vi "Decode Data.vi"(8 "Errors In":T1, 10 "Time Stamp":timestamp, 11 "Data Array":string[](array[string])) -> (0 "Errors Out":T1, 3 "logData Out":T2)   [LabVIEW 2014]
doc: "Decode hex data obtained from inverter boards into decimal measurements. DC bus voltage, current RMS, motor power, temp."
uses:
  TypeDefs/Errors.ctl
panel:
  in  "logData In":T3
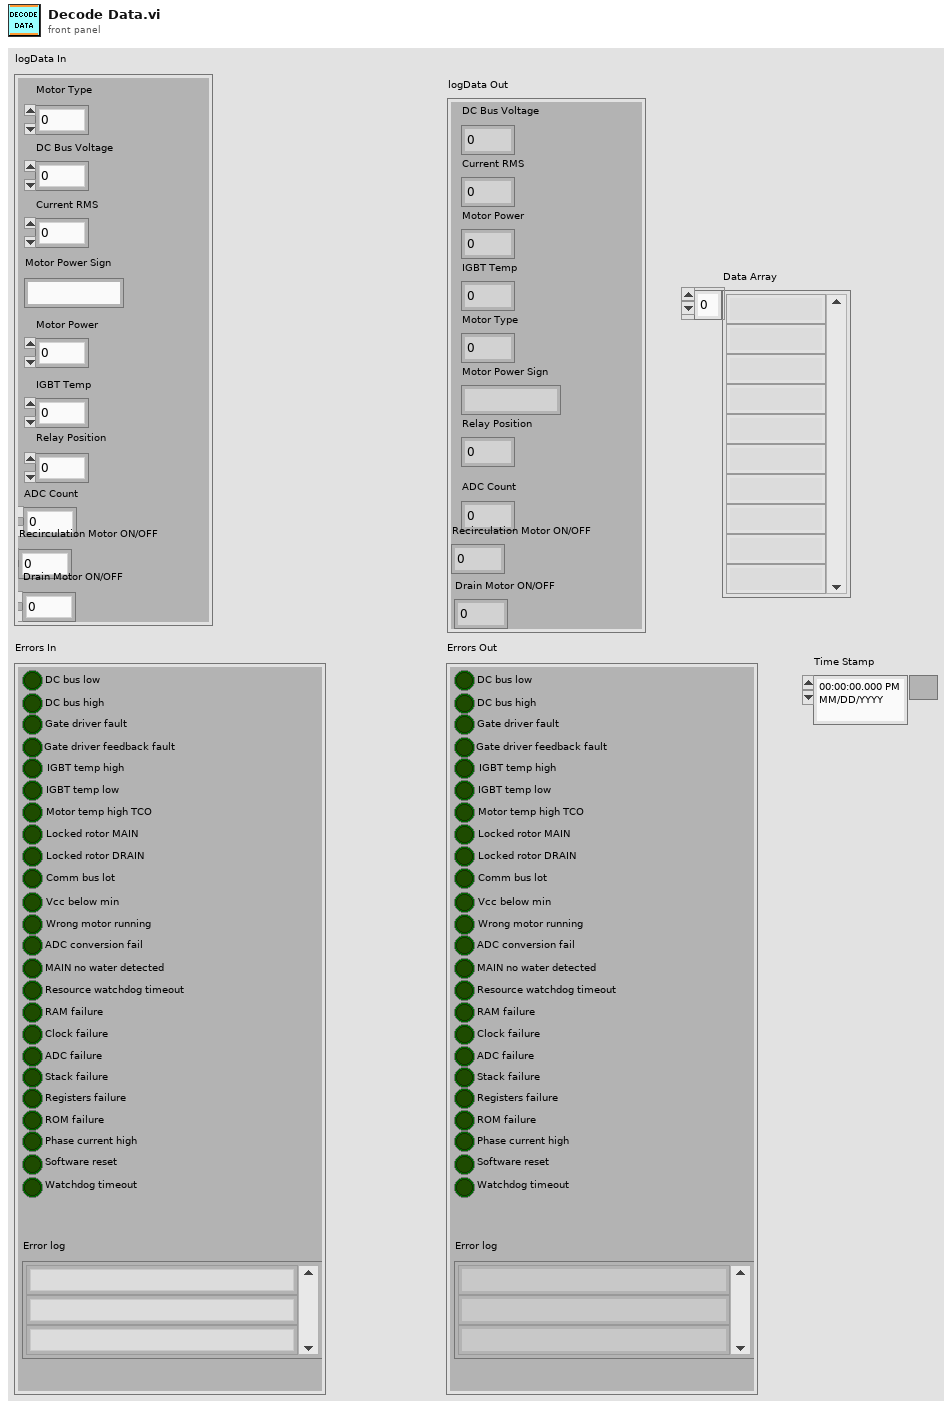
[diagram p1: front panel]
types:
  T1 = typedef "Errors.ctl" = cluster{"DC bus low":bool, "DC bus high":bool, "Gate driver fault":bool, "Gate driver feedback fault":bool, "IGBT temp high":bool, "IGBT temp low":bool, "Motor temp high TCO":bool, "Locked rotor MAIN":bool, "Locked rotor DRAIN":bool, "Comm bus lot":bool, "Vcc below min":bool, "Wrong motor running":bool, "ADC conversion fail":bool, "MAIN no water detected":bool, "Resource watchdog timeout":bool, "RAM failure":bool, "Clock failure":bool, "ADC failure":bool, "Stack failure":bool, "Registers failure":bool, "ROM failure":bool, "Phase current high":bool, "Software reset":bool, "Watchdog timeout":bool, "Error log":string[]}
  T2 = cluster{"DC Bus Voltage":dbl, "Current RMS":dbl, "Motor Power":dbl, "IGBT Temp":u16, "Motor Type":u16, "Motor Power Sign":string, "Relay Position":u16, "ADC Count":dbl, "Recirculation Motor ON/OFF":u16, "Drain Motor ON/OFF":u16}
  T3 = cluster{"DC Bus Voltage":dbl, "Current RMS":dbl, "Motor Power":dbl, "IGBT Temp":u32, "Motor Type":u16, "Motor Power Sign":string, "Relay Position":u16, "ADC Count":dbl, "Recirculation Motor ON/OFF":u32, "Drain Motor ON/OFF":u16}
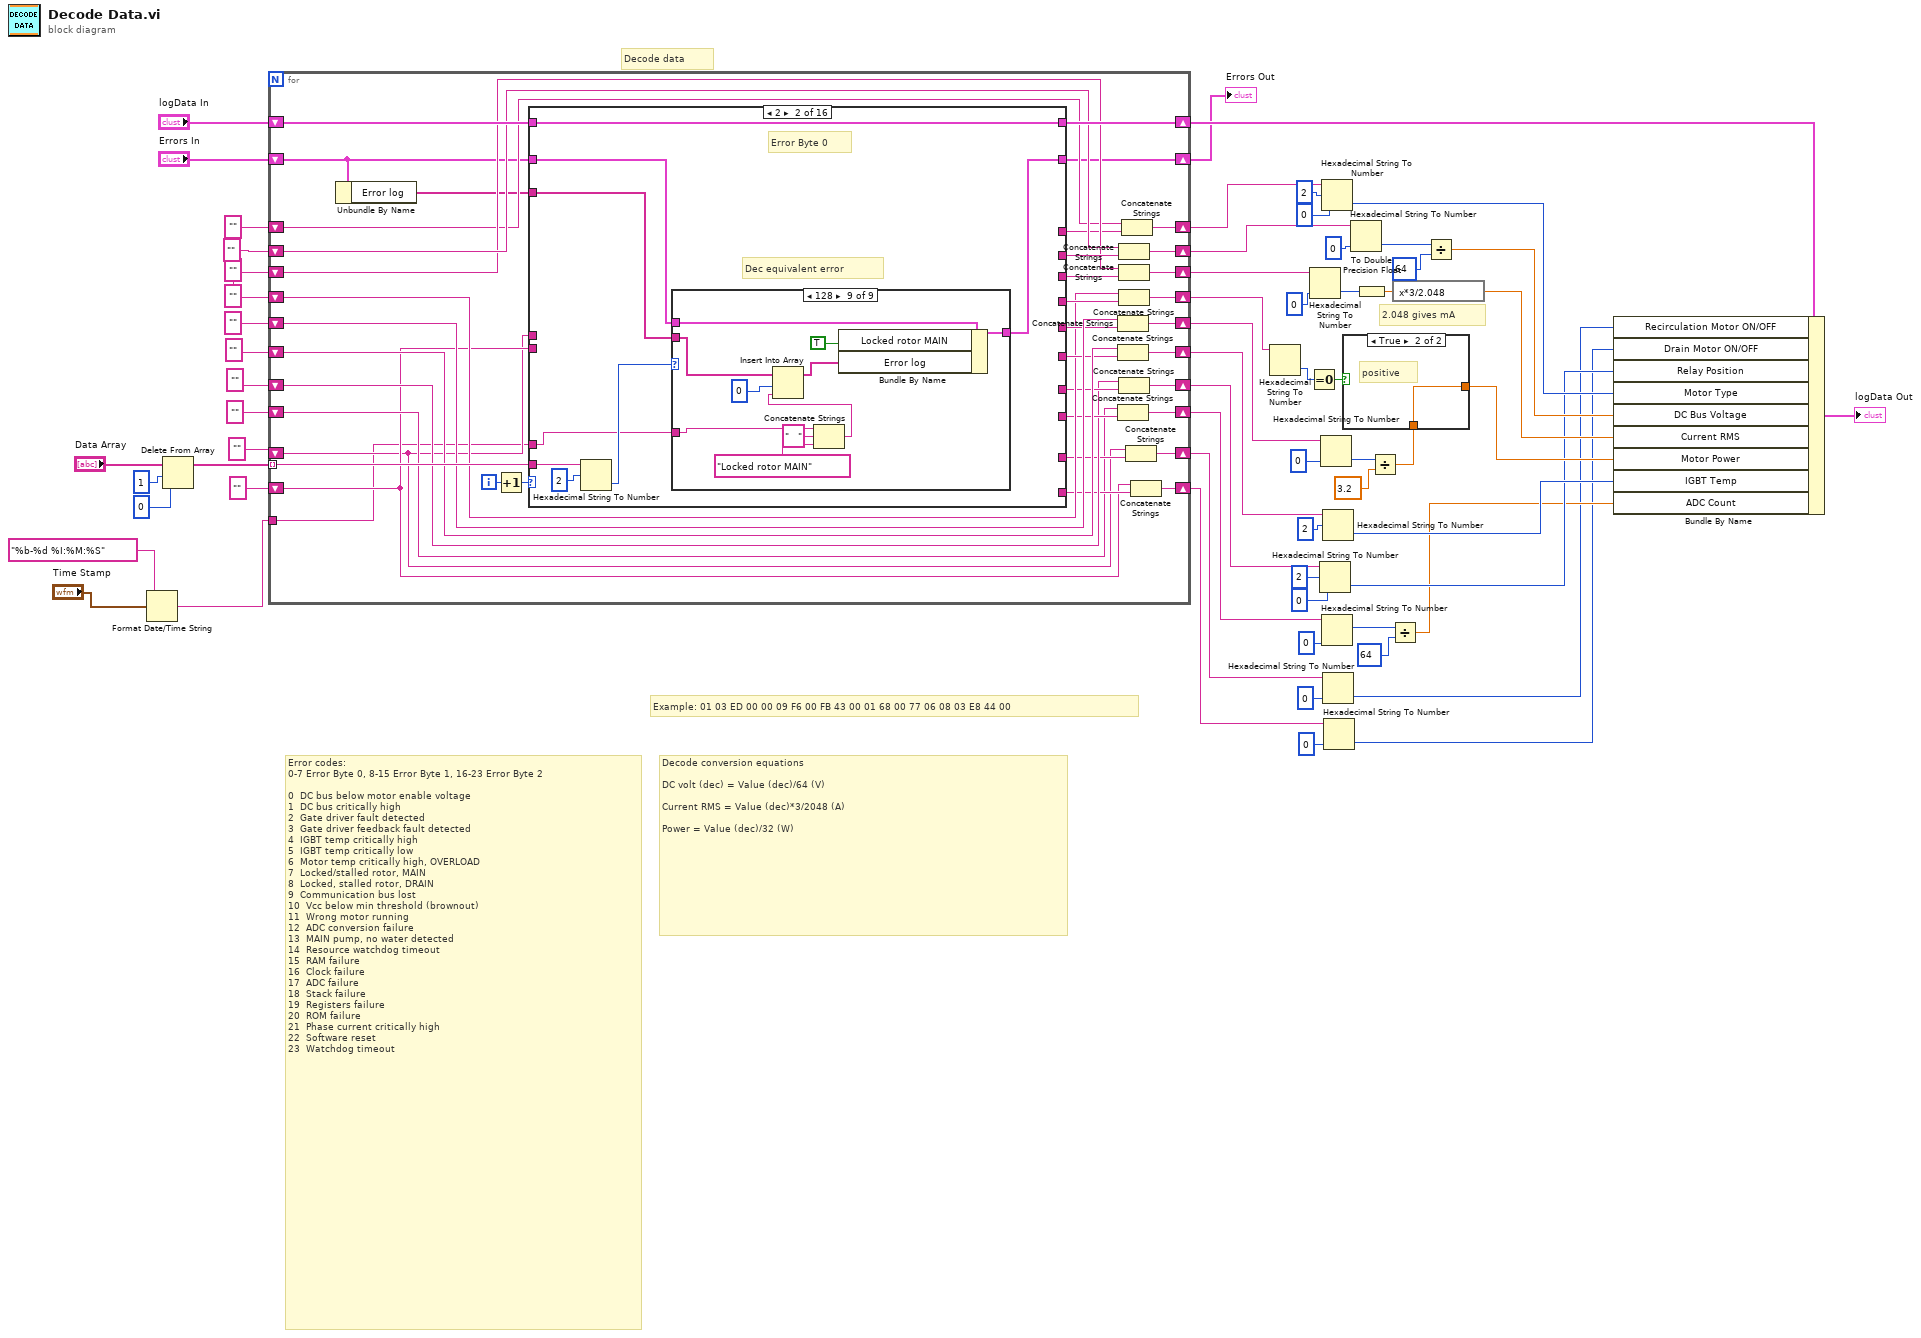
[diagram p0: block diagram]
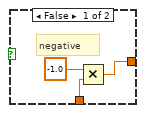
[diagram p2: hidden frame]
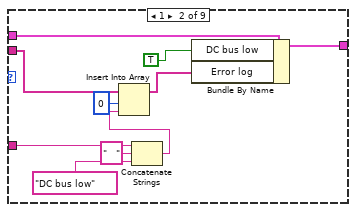
[diagram p5: hidden frame]
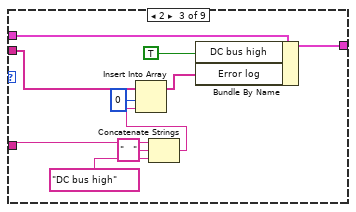
[diagram p6: hidden frame]
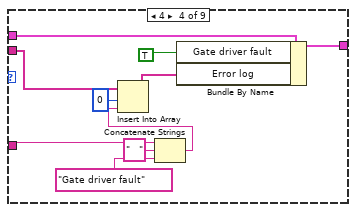
[diagram p7: hidden frame]
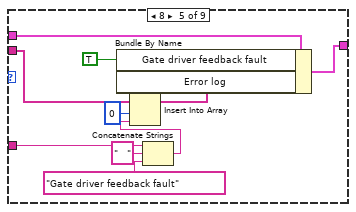
[diagram p8: hidden frame]
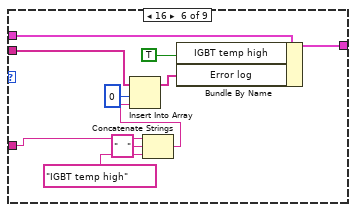
[diagram p9: hidden frame]
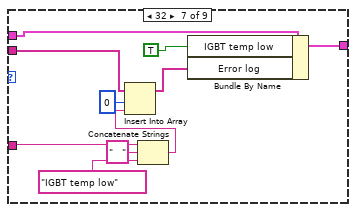
[diagram p10: hidden frame]
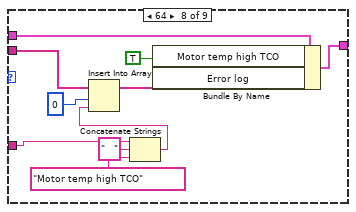
[diagram p11: hidden frame]
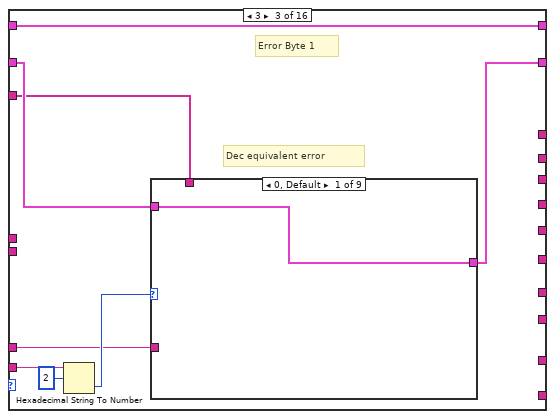
[diagram p12: hidden frame]
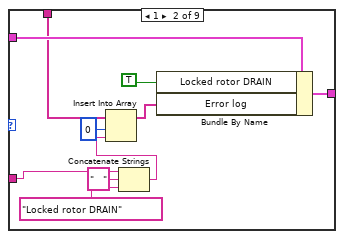
[diagram p13: hidden frame]
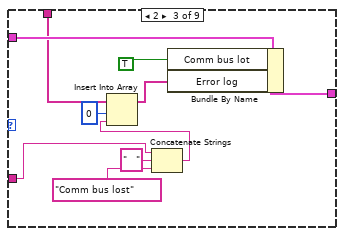
[diagram p14: hidden frame]
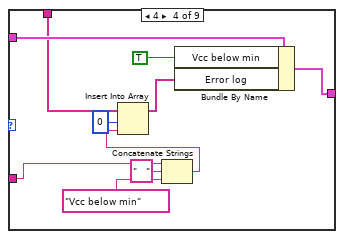
[diagram p15: hidden frame]
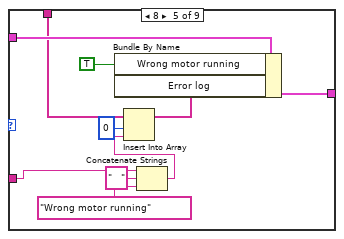
[diagram p16: hidden frame]
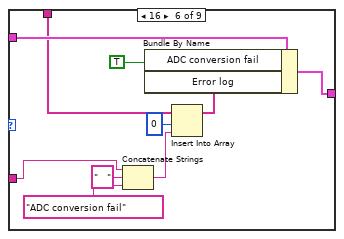
[diagram p17: hidden frame]
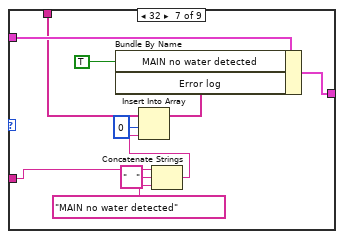
[diagram p18: hidden frame]
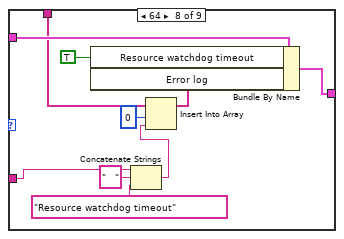
[diagram p19: hidden frame]
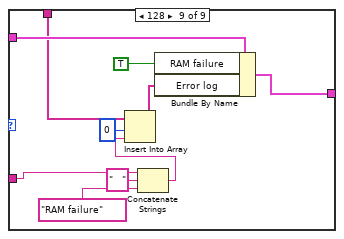
[diagram p20: hidden frame]
diagram:
  # "2.048 gives mA"
  # "Decode conversion equations\n\nDC volt (dec) = Value (dec)/64 (V)\n\nCurrent RMS = Value (dec)*3/2048 (A)\n\nPower = Value (dec)/32 (W)"
  # "Error codes:\n0-7 Error Byte 0, 8-15 Error Byte 1, 16-23 Error Byte 2\n\n0  DC bus below motor enable voltage\n1  DC bus critically high\n2  Gate driver fault detected\n3  Gate driver feedback fault detected\n4  IGBT temp critically high\n5  IGBT temp critically low\n6  Motor temp critically high, OVERLOAD\n7  Locked/stalled rotor, MAIN\n8  Locked, stalled rotor, DRAIN\n9  Communication bus lost\n10  Vcc below min threshold (brownout)\n11  Wrong motor running\n12  ADC conversion failure\n13  MAIN pump, no water detected\n14  Resource watchdog timeout\n15  RAM failure \n16  Clock failure\n17  ADC failure\n18  Stack failure\n19  Registers failure\n20  ROM failure\n21  Phase current critically high\n22  Software reset\n23  Watchdog timeout"
  # "Example: 01 03 ED 00 00 09 F6 00 FB 43 00 01 68 00 77 06 08 03 E8 44 00"
  # "Decode data"
  n1 = Format Date/Time String(time format string (%c)="%b-%d %I:%M:%S", seconds (now)="Time Stamp") -> (date/time string=w1:string)  [unwired: 1 in]
  n2 = Delete From Array(array="Data Array", length=1, index=0) -> (array with subset deleted=w4:string[])  [unwired: 1 out]
  n3 = for {
    tunnel: w4 -> [w102] mode=indexing
    shift-right: [w100] -> w52
    shift-left: "logData In" -> [w99]
    shift-right: [w95] -> w54
    shift-left: "" -> [w97]
    shift-right: [w92] -> w58
    shift-left: "" -> [w94]
    shift-right: [w89] -> w61
    shift-left: "" -> [w91]
    shift-right: [w86] -> w63
    shift-left: "" -> [w88]
    shift-right: [w83] -> w38
    shift-left: "" -> [w84]
    shift-right: [w81] -> w32
    shift-left: "" -> [w79]
    shift-right: [w82] -> w37
    shift-left: "Errors In" -> [w66]
    shift-right: [w78] -> w26
    shift-left: "" -> [w74]
    shift-right: [w75] -> w20
    shift-left: "" -> [w69]
    shift-right: [w72] -> w15
    shift-left: "" -> [w67]
    shift-right: [w73] -> w14
    shift-left: "" -> [w68]
    tunnel: w1 -> [w64]
    i -> [w101]
    n4 = Unbundle By Name(w66) -> ("Error log"=w65:string[])
    n5 = Increment(x=w101) -> (x+1=w98:i32)
    n6 = case shown="2" w98 {
      tunnel: w102 -> [w104 w113 w202 w290 w376 w380 w384 w389 w394 w400 w404 w409 w411 w415 w420 w429]
      tunnel: w99 -> [w105 w108 w198 w287 w377 w382 w387 w392 w397 w402 w407 w410 w413 w418 w423 w433]
      tunnel: [w105 w108 w198 w287 w377 w382 w387 w392 w397 w402 w407 w410 w413 w418 w423 w433] -> w100
      tunnel: [_ _ _ _ w375 w379 _ _ _ _ _ _ _ _ _ _] -> w96
      tunnel: [_ _ _ _ _ _ w385 w390 _ _ _ _ _ _ _ _] -> w93
      tunnel: [_ _ _ _ _ _ _ _ _ w398 w405 _ _ _ _ _] -> w90
      tunnel: [_ _ _ _ _ _ _ _ _ _ _ w409 _ _ _ _] -> w87
      tunnel: [w104 _ _ _ _ _ _ _ _ _ _ _ _ _ _ _] -> w85
      tunnel: w66 -> [w103 w110 w199 w288 w373 w378 w383 w388 w396 w399 w403 w408 w412 w417 w422 w432]
      tunnel: [w103 w109 w197 w286 w373 w378 w383 w388 w396 w399 w403 w408 w412 w417 w422 w432] -> w82
      tunnel: [_ _ _ _ _ _ _ _ w393 _ _ _ _ _ _ _] -> w80
      tunnel: [_ _ _ _ _ _ _ _ _ _ _ _ w411 _ _ _] -> w77
      tunnel: [_ _ _ _ _ _ _ _ _ _ _ _ _ w414 w419 _] -> w76
      tunnel: [_ _ _ _ _ _ _ _ _ _ _ _ _ _ _ w427] -> w70
      tunnel: [_ _ _ _ _ _ _ _ _ _ _ _ _ _ _ w426] -> w71
      tunnel: w67 -> [_ _ _ _ _ _ _ _ _ _ _ _ _ _ _ w425]
      tunnel: w68 -> [_ _ _ _ _ _ _ _ _ _ _ _ _ _ _ w424]
      tunnel: w65 -> [_ w106 w196 w284 _ _ _ _ _ _ _ _ _ _ _ _]
      tunnel: w64 -> [_ w107 w195 w285 _ _ _ _ _ _ _ _ _ _ _ _]
      frame 1, Default {
        # "Motor type"
      }
      frame 2 {
        # "Dec equivalent error"
        # "Error Byte 0"
        n7 = Hexadecimal String To Number(string=w113, offset=2) -> (number=w111:u32)  [unwired: 1 in, 1 out]
        n8 = case shown="128" w111 {
          tunnel: w110 -> [w114 w122 w134 w144 w153 w163 w173 w183 w193]
          tunnel: [w114 w123 w133 w143 w152 w162 w172 w182 w192] -> w109
          tunnel: w107 -> [_ w118 w128 w138 w148 w158 w168 w178 w188]
          tunnel: w106 -> [_ w117 w127 w137 w147 w157 w166 w176 w187]
          frame 0, Default {
          }
          frame 1 {
            n9 = Concatenate Strings(w118, "   " ("string"), "DC bus low") -> (w121:string)
            n10 = Insert Into Array(array=w117, index=0, new element=w121) -> (w116:string[])
            n11 = Bundle By Name(cluster=w122, "DC bus low"=TRUE, "Error log"=w116) -> (w123:T1)
          }
          frame 2 {
            n12 = Concatenate Strings(w128, "   " ("string"), "DC bus high") -> (w131:string)
            n13 = Insert Into Array(array=w127, index=0, new element=w131) -> (w126:string[])
            n14 = Bundle By Name(cluster=w134, "DC bus high"=TRUE ("Errors.Locked rotor DRAIN"), "Error log"=w126) -> (w133:T1)
          }
          frame 4 {
            n15 = Concatenate Strings(w138, "   " ("string"), "Gate driver fault") -> (w141:string)
            n16 = Insert Into Array(array=w137, index=0, new element=w141) -> (w136:string[])
            n17 = Bundle By Name(cluster=w144, "Gate driver fault"=TRUE ("Errors.Vcc below min"), "Error log"=w136) -> (w143:T1)
          }
          frame 8 {
            n18 = Concatenate Strings(w148, "   " ("string"), "Gate driver feedback fault") -> (w151:string)
            n19 = Insert Into Array(array=w147, index=0, new element=w151) -> (w146:string[])
            n20 = Bundle By Name(cluster=w153, "Gate driver feedback fault"=TRUE ("Errors.Vcc below min"), "Error log"=w146) -> (w152:T1)
          }
          frame 16 {
            n21 = Concatenate Strings(w158, "   " ("string"), "IGBT temp high") -> (w161:string)
            n22 = Insert Into Array(array=w157, index=0, new element=w161) -> (w156:string[])
            n23 = Bundle By Name(cluster=w163, "IGBT temp high"=TRUE ("Errors.Vcc below min"), "Error log"=w156) -> (w162:T1)
          }
          frame 32 {
            n24 = Concatenate Strings(w168, "   " ("string"), "IGBT temp low") -> (w171:string)
            n25 = Insert Into Array(array=w166, index=0, new element=w171) -> (w167:string[])
            n26 = Bundle By Name(cluster=w173, "IGBT temp low"=TRUE ("Errors.Vcc below min"), "Error log"=w167) -> (w172:T1)
          }
          frame 64 {
            n27 = Concatenate Strings(w178, "   " ("string"), "Motor temp high TCO") -> (w181:string)
            n28 = Insert Into Array(array=w176, index=0, new element=w181) -> (w177:string[])
            n29 = Bundle By Name(cluster=w183, "Motor temp high TCO"=TRUE ("Errors.Vcc below min"), "Error log"=w177) -> (w182:T1)
          }
          frame 128 {
            n30 = Concatenate Strings(w188, "   " ("string"), "Locked rotor MAIN") -> (w186:string)
            n31 = Insert Into Array(array=w187, index=0, new element=w186) -> (w185:string[])
            n32 = Bundle By Name(cluster=w193, "Locked rotor MAIN"=TRUE ("Errors.Vcc below min"), "Error log"=w185) -> (w192:T1)
          }
        }
      }
      frame 3 {
        # "Dec equivalent error"
        # "Error Byte 1"
        n33 = Hexadecimal String To Number(string=w202, offset=2) -> (number=w200:u32)  [unwired: 1 in, 1 out]
        n34 = case shown="0, Default" w200 {
          tunnel: w199 -> [w203 w211 w223 w233 w242 w252 w262 w272 w282]
          tunnel: [w203 w212 w222 w232 w241 w251 w261 w271 w281] -> w197
          tunnel: w196 -> [_ w209 w216 w226 w235 w246 w256 w266 w276]
          tunnel: w195 -> [_ w208 w217 w227 w237 w247 w257 w267 w277]
          frame 0, Default {
          }
          frame 1 {
            n35 = Concatenate Strings(w208, "   " ("string"), "Locked rotor DRAIN") -> (w207:string)
            n36 = Insert Into Array(array=w209, index=0, new element=w207) -> (w210:string[])
            n37 = Bundle By Name(cluster=w211, "Locked rotor DRAIN"=TRUE ("DC bus low"), "Error log"=w210) -> (w212:T1)
          }
          frame 2 {
            n38 = Concatenate Strings(w217, "   " ("string"), "Comm bus lost") -> (w220:string)
            n39 = Insert Into Array(array=w216, index=0, new element=w220) -> (w215:string[])
            n40 = Bundle By Name(cluster=w223, "Comm bus lot"=TRUE ("Errors.Locked rotor DRAIN"), "Error log"=w215) -> (w222:T1)
          }
          frame 4 {
            n41 = Concatenate Strings(w227, "   " ("string"), "Vcc below min") -> (w230:string)
            n42 = Insert Into Array(array=w226, index=0, new element=w230) -> (w225:string[])
            n43 = Bundle By Name(cluster=w233, "Vcc below min"=TRUE ("Errors.Vcc below min"), "Error log"=w225) -> (w232:T1)
          }
          frame 8 {
            n44 = Concatenate Strings(w237, "   " ("string"), "Wrong motor running") -> (w240:string)
            n45 = Insert Into Array(array=w235, index=0, new element=w240) -> (w236:string[])
            n46 = Bundle By Name(cluster=w242, "Wrong motor running"=TRUE ("Errors.Vcc below min"), "Error log"=w236) -> (w241:T1)
          }
          frame 16 {
            n47 = Concatenate Strings(w247, "   " ("string"), "ADC conversion fail") -> (w250:string)
            n48 = Insert Into Array(array=w246, index=0, new element=w250) -> (w245:string[])
            n49 = Bundle By Name(cluster=w252, "ADC conversion fail"=TRUE ("Errors.Vcc below min"), "Error log"=w245) -> (w251:T1)
          }
          frame 32 {
            n50 = Concatenate Strings(w257, "   " ("string"), "MAIN no water detected") -> (w260:string)
            n51 = Insert Into Array(array=w256, index=0, new element=w260) -> (w255:string[])
            n52 = Bundle By Name(cluster=w262, "MAIN no water detected"=TRUE ("Errors.Vcc below min"), "Error log"=w255) -> (w261:T1)
          }
          frame 64 {
            n53 = Concatenate Strings(w267, "   " ("string"), "Resource watchdog timeout") -> (w270:string)
            n54 = Insert Into Array(array=w266, index=0, new element=w270) -> (w265:string[])
            n55 = Bundle By Name(cluster=w272, "Resource watchdog timeout"=TRUE ("Errors.Vcc below min"), "Error log"=w265) -> (w271:T1)
          }
          frame 128 {
            n56 = Concatenate Strings(w277, "   " ("string"), "RAM failure") -> (w280:string)
            n57 = Insert Into Array(array=w276, index=0, new element=w280) -> (w275:string[])
            n58 = Bundle By Name(cluster=w282, "RAM failure"=TRUE ("Errors.Vcc below min"), "Error log"=w275) -> (w281:T1)
          }
        }
      }
      frame 4 {
        # "Error Byte 2"
        # "Dec equivalent error"
        n59 = Hexadecimal String To Number(string=w290, offset=2) -> (number=w289:u32)  [unwired: 1 in, 1 out]
        n60 = case shown="0, Default" w289 {
          tunnel: w288 -> [w292 w300 w312 w322 w331 w341 w351 w361 w371]
          tunnel: [w292 w301 w311 w321 w330 w340 w350 w360 w370] -> w286
          tunnel: w285 -> [_ w295 w305 w315 w325 w335 w345 w355 w365]
          tunnel: w284 -> [_ w294 w304 w314 w324 w334 w344 w354 w364]
          frame 0, Default {
          }
          frame 1 {
            n61 = Concatenate Strings(w295, "   " ("string"), "Clock failure") -> (w296:string)
            n62 = Insert Into Array(array=w294, index=0, new element=w296) -> (w293:string[])
            n63 = Bundle By Name(cluster=w300, "Clock failure"=TRUE ("DC bus low"), "Error log"=w293) -> (w301:T1)
          }
          frame 2 {
            n64 = Concatenate Strings(w305, "   " ("string"), "ADC failure") -> (w306:string)
            n65 = Insert Into Array(array=w304, index=0, new element=w306) -> (w303:string[])
            n66 = Bundle By Name(cluster=w312, "ADC failure"=TRUE ("Errors.Locked rotor DRAIN"), "Error log"=w303) -> (w311:T1)
          }
          frame 4 {
            n67 = Concatenate Strings(w315, "   " ("string"), "Stack failure") -> (w316:string)
            n68 = Insert Into Array(array=w314, index=0, new element=w316) -> (w313:string[])
            n69 = Bundle By Name(cluster=w322, "Stack failure"=TRUE ("Errors.Vcc below min"), "Error log"=w313) -> (w321:T1)
          }
          frame 8 {
            n70 = Concatenate Strings(w325, "   " ("string"), "Registers failure") -> (w326:string)
            n71 = Insert Into Array(array=w324, index=0, new element=w326) -> (w323:string[])
            n72 = Bundle By Name(cluster=w331, "Registers failure"=TRUE ("Errors.Vcc below min"), "Error log"=w323) -> (w330:T1)
          }
          frame 16 {
            n73 = Concatenate Strings(w335, "   " ("string"), "ROM failure") -> (w336:string)
            n74 = Insert Into Array(array=w334, index=0, new element=w336) -> (w333:string[])
            n75 = Bundle By Name(cluster=w341, "ROM failure"=TRUE ("Errors.Vcc below min"), "Error log"=w333) -> (w340:T1)
          }
          frame 32 {
            n76 = Concatenate Strings(w345, "   " ("string"), "Phase current high") -> (w346:string)
            n77 = Insert Into Array(array=w344, index=0, new element=w346) -> (w343:string[])
            n78 = Bundle By Name(cluster=w351, "Phase current high"=TRUE ("Errors.Vcc below min"), "Error log"=w343) -> (w350:T1)
          }
          frame 64 {
            n79 = Concatenate Strings(w355, "   " ("string"), "Software reset") -> (w356:string)
            n80 = Insert Into Array(array=w354, index=0, new element=w356) -> (w353:string[])
            n81 = Bundle By Name(cluster=w361, "Software reset"=TRUE ("Errors.Vcc below min"), "Error log"=w353) -> (w360:T1)
          }
          frame 128 {
            n82 = Concatenate Strings(w365, "   " ("string"), "Watchdog timeout") -> (w366:string)
            n83 = Insert Into Array(array=w364, index=0, new element=w366) -> (w363:string[])
            n84 = Bundle By Name(cluster=w371, "Watchdog timeout"=TRUE ("Errors.Vcc below min"), "Error log"=w363) -> (w370:T1)
          }
        }
      }
      frame 5 {
        # "DC Bus Voltage MSB"
        n85 = String Subset(string=w376, offset (0)=2) -> (substring=w375:string)  [unwired: 1 in]
      }
      frame 6 {
        # "DC Bus Voltage LSB"
        n86 = String Subset(string=w380, offset (0)=2) -> (substring=w379:string)  [unwired: 1 in]
      }
      frame 7 {
        # "Current RMS MSB"
        n87 = String Subset(string=w384, offset (0)=2) -> (substring=w385:string)  [unwired: 1 in]
      }
      frame 8 {
        # "Current RMS LSB"
        n88 = String Subset(string=w389, offset (0)=2) -> (substring=w390:string)  [unwired: 1 in]
      }
      frame 9 {
        # "0x00 positive\n0x01 negative"
        # "Motor Power Sign"
        n89 = String Subset(string=w394, offset (0)=2) -> (substring=w393:string)  [unwired: 1 in]
      }
      frame 10 {
        # "Motor Power MSB"
        n90 = String Subset(string=w400, offset (0)=2) -> (substring=w398:string)  [unwired: 1 in]
      }
      frame 11 {
        # "Motor Power LSB"
        n91 = String Subset(string=w404, offset (0)=2) -> (substring=w405:string)  [unwired: 1 in]
      }
      frame 12 {
        # "IGBT Temp"
      }
      frame 13 {
        # "Relay Position State"
      }
      frame 14 {
        # "Relay Position ADC Count MSB"
        n92 = String Subset(string=w415, offset (0)=2) -> (substring=w414:string)  [unwired: 1 in]
      }
      frame 15 {
        # "Relay Position ADC Count LSB"
        n93 = String Subset(string=w420, offset (0)=2) -> (substring=w419:string)  [unwired: 1 in]
      }
      frame 16 {
        # "ALT Test Profile Index"
        n94 = Hexadecimal String To Number(string=w429, offset=2, default (0uL)=u32 0 ("default (0 U32)")) -> (number=w428:u32)  [unwired: 1 out]
        n95 = case shown="2, 6, 10, 14, 18, 22, 26" w428 {
          tunnel: [w434 w436 "01" "00"] -> w427
          tunnel: w424 -> [w434 w436 _ _]
          tunnel: w425 -> [_ _ w438 w440]
          tunnel: ["01" "00" w438 w440] -> w426
          frame 0, 4, 8, 12, 16, 20, 24, 28, Default {
            # "Recirculation motor ON"
          }
          frame 1, 5, 9, 13, 17, 21, 25, 29 {
            # "Recirculation motor OFF"
          }
          frame 2, 6, 10, 14, 18, 22, 26 {
            # "drain motor ON"
          }
          frame 3, 7, 11, 15, 19, 23, 27 {
            # "drain motor OFF"
          }
        }
      }
    }
    n96 = Concatenate Strings(w91, w90) -> (w89:string)
    n97 = Concatenate Strings(w88, w87) -> (w86:string)
    n98 = Concatenate Strings(w69, w76) -> (w75:string)
    n99 = Concatenate Strings(w97, w96) -> (w95:string)
    n100 = Concatenate Strings(w94, w93) -> (w92:string)
    n101 = Concatenate Strings(w79, w80) -> (w81:string)
    n102 = Concatenate Strings(w74, w77) -> (w78:string)
    n103 = Concatenate Strings(w84, w85) -> (w83:string)
    n104 = Concatenate Strings(w67, w71) -> (w72:string)
    n105 = Concatenate Strings(w68, w70) -> (w73:string)
  }
  "Errors Out" <- w37
  n106 = Hexadecimal String To Number(string=w32) -> (number=w33:u32)  [unwired: 2 in, 1 out]
  n107 = Equal To 0?(x=w33) -> (x = 0?=w31:bool)
  n108 = Hexadecimal String To Number(string=w58, default (0uL)=u16 0 ("default (0 U32)")) -> (number=w35:u16)  [unwired: 1 in, 1 out]
  n109 = Hexadecimal String To Number(string=w26, offset=2, default (0uL)=u32 0 ("default (0 U32)")) -> (number=w25:u32)  [unwired: 1 out]
  n110 = Hexadecimal String To Number(string=w61, default (0uL)=u16 0 ("default (0 U32)")) -> (number=w50:u16)  [unwired: 1 in, 1 out]
  n111 = Hexadecimal String To Number(string=w38, offset=2, default (0uL)=u32 0 ("default (0 U32)")) -> (number=w39:u32)  [unwired: 1 out]
  n112 = Hexadecimal String To Number(string=w20, default (0uL)=u16 0 ("default (0 U32)")) -> (number=w21:u16)  [unwired: 1 in, 1 out]
  n113 = Hexadecimal String To Number(string=w63, offset=2) -> (number=w40:u32)  [unwired: 1 in, 1 out]
  n114 = Hexadecimal String To Number(string=w15, default (0uL)=u32 0 ("default (0 U32)")) -> (number=w13:u32)  [unwired: 1 in, 1 out]
  n115 = Hexadecimal String To Number(string=w14, default (0uL)=u32 0 ("default (0 U32)")) -> (number=w12:u32)  [unwired: 1 in, 1 out]
  n116 = Hexadecimal String To Number(string=w54, default (0uL)=u16 0 ("default (0 U32)")) -> (number=w49:u16)  [unwired: 1 in, 1 out]
  n117 = To Double Precision Float(number=w35) -> (double precision float=w47:dbl)
  n118 = Divide(x=w50, y=3.2) -> (x/y=w10:dbl)
  n119 = case shown="True" w31 {
    tunnel: w10 -> [w443 w445]
    tunnel: [w442 w445] -> w36
    frame False {
      # "negative"
      n120 = Multiply(x=-1.0, y=w443) -> (x*y=w442:dbl)
    }
    frame True {
      # "positive"
    }
  }
  n121 = Divide(x=w21, y=u16 64) -> (x/y=w19:dbl)
  n122 = expression code="x*3/2.048"(w47) -> (w45:dbl)
  n123 = Divide(x=w49, y=u16 64) -> (x/y=w46:dbl)
  n124 = Bundle By Name(cluster=w52, "Recirculation Motor ON/OFF"=w13, "Drain Motor ON/OFF"=w12, "Relay Position"=w25, "Motor Type"=w39, "DC Bus Voltage"=w46, "Current RMS"=w45, "Motor Power"=w36, "IGBT Temp"=w40, "ADC Count"=w19) -> (→"logData Out":T3)
